vi "836_CameraStartStopCount.vi"(8 "error in (no error)":errorcluster, 10 "Action":enum16{"Start", "Stop"}(ring), 11 "Camera Address Out":string) -> (0 "error out":errorcluster)   [LabVIEW 2015]
uses:
  <vilib>/vision/driver/NI_Vision_Acquisition_Software.lvlib
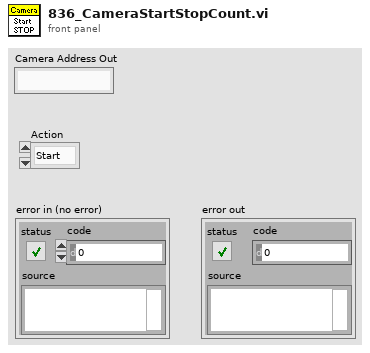
[diagram p1: front panel]
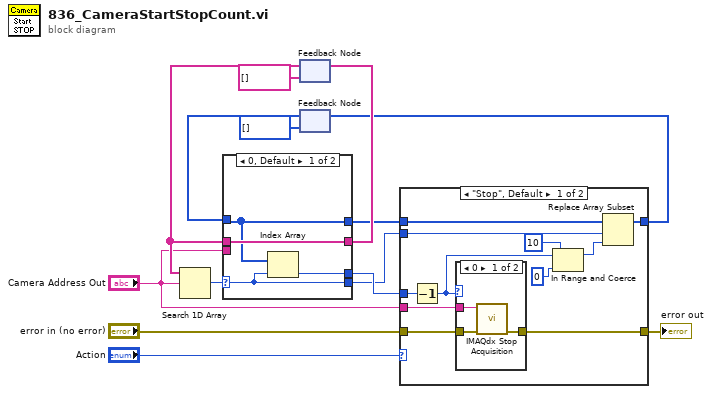
[diagram p0: block diagram]
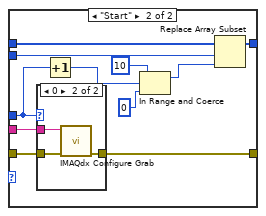
[diagram p3: hidden frame]
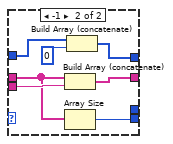
[diagram p5: hidden frame]
diagram:
  n1 = feedback #1(string[] []) -> (w11:string[])
  n2 = Search 1D Array(1D array=w11, element="Camera Address Out") -> (index of element=w12:i32)  [unwired: 1 in]
  n3 = feedback #2(i32[] []) -> (w10:i32[])
  n4 = case shown="0, Default" w12 {
    selector: w12 -> [w15 _]
    tunnel: w11 -> [w18 w20]
    tunnel: w10 -> [w17 w25]
    tunnel: [w17 w21] -> w2
    tunnel: [w18 w23] -> w9
    tunnel: "Camera Address Out" -> [_ w24]
    tunnel: [w16 _] -> w6
    tunnel: [w15 w19] -> w3
    frame 0, Default {
      n5 = Index Array(array=w17, index=w15) -> (element=w16:i32)
    }
    frame -1 {
      n6 = Build Array (concatenate)(w20, w24) -> (w23:string[])
      n7 = Array Size(array=w20) -> (size(s)=w19:i32)
      n8 = Build Array (concatenate)(w25, 0) -> (w21:i32[])
    }
  }
  n9 = feedback-in #1(w9) -> ()
  n10 = case shown="\"Stop\", Default" "Action" {
    tunnel: [w31 w51] -> w14
    tunnel: "error in (no error)" -> [w32 w50]
    tunnel: "Camera Address Out" -> [w30 w49]
    tunnel: w6 -> [w33 w46]
    tunnel: w3 -> [w34 w47]
    tunnel: w2 -> [w35 w48]
    tunnel: [w36 w45] -> w1
    frame "Stop", Default {
      n11 = Decrement(x=w33) -> (x-1=w27:i32)
      n12 = case shown="0" w27 {
        tunnel: w32 -> [w39 w40]
        tunnel: [w38 w40] -> w31
        tunnel: w30 -> [w37 _]
        frame 0 {
          n13 = call <vilib>:"IMAQdx Stop Acquisition.vi"("error in"=w39, "Session In"=w37) -> ("error out"=w38:errorcluster)  [unwired: 8 in, 1 out]
        }
        frame 1, Default {
        }
      }
      n14 = In Range and Coerce(upper limit=10 ("lower limit"), x=w27, lower limit=0) -> (coerced(x)=w26:i32)  [unwired: 1 out]
      n15 = Replace Array Subset(array=w35, new element=w26, index=w34) -> (w36:i32[])
    }
    frame "Start" {
      n16 = case shown="0" w46 {
        tunnel: [w52 w55] -> w51
        tunnel: w50 -> [w52 w54]
        tunnel: w49 -> [_ w53]
        frame Default {
        }
        frame 0 {
          n17 = call <vilib>:"IMAQdx Configure Grab.vi"("error in"=w54, "Session In"=w53) -> ("error out"=w55:errorcluster)  [unwired: 8 in, 1 out]
        }
      }
      n18 = Increment(x=w46) -> (x+1=w42:i32)
      n19 = In Range and Coerce(upper limit=10 ("lower limit"), x=w42, lower limit=0) -> (coerced(x)=w41:i32)  [unwired: 1 out]
      n20 = Replace Array Subset(array=w48, new element=w41, index=w47) -> (w45:i32[])
    }
  }
  "error out" <- w14
  n21 = feedback-in #2(w1) -> ()
